vi "Get Motor Power.vi"(11 "Motor refnum name":string) -> (3 "Max Power":dbl)   [LabVIEW 2013]
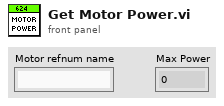
[diagram p1: front panel]
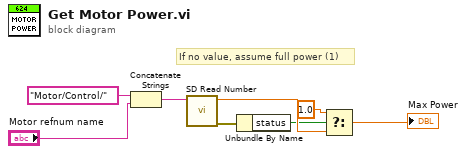
[diagram p0: block diagram]
diagram:
  # "If no value, assume full power (1)"
  n1 = Concatenate Strings("Motor/Control/" ("string"), "Motor refnum name") -> (w1:string)
  n2 = call <vilib>:"SD Read Number.vi"("Name"=w1) -> ("error out"=w4:errorcluster, "Numeric"=w7:dbl)  [unwired: 8 in, 1 out]
  n3 = Unbundle By Name(w4) -> ("status"=w5:bool)
  n4 = Select(t=1.0, s=w5, f=w7) -> (s? t:f=→"Max Power":dbl)
